vi "moving average.vi"(7 "length":i32=20, 8 "Numeric Array":dbl[](array[numeric])) -> (0 "Average Array":dbl[](array[numeric]))   [LabVIEW 2018]
uses:
  <vilib>/Analysis/baseanly.llb/Mean (DBL).vi
  <vilib>/Analysis/NI_AALBase.lvlib
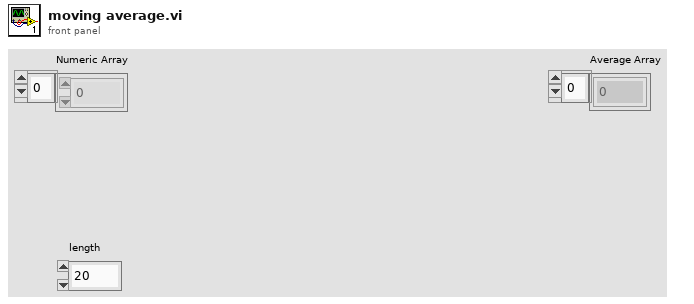
[diagram p1: front panel]
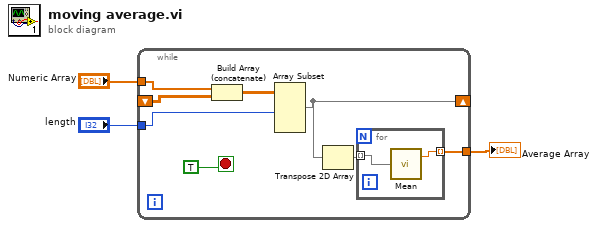
[diagram p0: block diagram]
diagram:
  n1 = while {
    tunnel: "Numeric Array" -> [w11]
    tunnel: "length" -> [w9]
    shift-right: [w7] -> _
    shift-left: _ -> [w8]
    tunnel: [w5] -> w1
    stop <- TRUE stop-if-true
    n2 = Build Array (concatenate)(w11, w8) -> (w10:dbl[][])
    n3 = Array Subset(array=w10, length (row)=w9) -> (w7:dbl[][])  [unwired: 3 in]
    n4 = Transpose 2D Array(2D array=w7) -> (transposed array=w6:dbl[][])
    n5 = for {
      tunnel: w6 -> [w13] mode=indexing
      tunnel: [w12] -> w5 mode=indexing
      n6 = call-poly <vilib>:"Mean.vi"("X"=w13) -> ("mean"=w12:dbl)  [unwired: 1 out]
    }
  }
  "Average Array" <- w1
